vi "Handle Error.vi"(8 "error in (no error)":errorcluster, 11 "Sim Sensor Interface Actor in":refnum<class "Sim Sensor Interface Actor.lvclass">) -> (0 "error out":errorcluster, 2 "stop actor?":bool=TRUE, 3 "Sim Sensor Interface Actor out":refnum<class "Sim Sensor Interface Actor.lvclass">)   [LabVIEW 2022 SP3, in "Sim Sensor Interface Actor.lvlib" / "Sim Sensor Interface Actor.lvclass"]
doc: "(<B>Filename</B>: Actor Framework.lvlib:Actor.lvclass:Handle Error.vi)\n\nDefines how the actor handles an error that occurred while processing a message.\n\nBy default, this method does nothing except stop the actor. This method also treats error code 43 (coming from <B>error in</B>) as a sign that the actor shut down normally. In this situation, the Handle Error method does not return the error on <B>error out</B>, meaning the actor's caller will not receive it. All other error codes will be returned on <B>error out</B>.\n\nA descendant class may override this method to change this behavior."
uses:
  Sim Sensor Interface Actor.lvclass
  C:/Program Files/National Instruments/LabVIEW 2022/vi.lib/ActorFramework/Actor/Actor.lvclass
  Elevator Controller/Elevator Controller/States -Enum.ctl
  <vilib>/ActorFramework/Actor/Actor.lvclass/Actor.ctl
  Elevator Controller/Elevator Controller Messages/Centralize Error Msg/Centralize Error Msg.lvclass/Centralize Error Msg.ctl
  <vilib>/ActorFramework/Message Enqueuer/Message Enqueuer.lvclass/Message Enqueuer.ctl
  Elevator Controller/Elevator Controller Messages/Set State Msg/Set State Msg.lvclass/Set State Msg.ctl
  <vilib>/ActorFramework/Message Enqueuer/Enqueue.vi
  Elevator Controller/Elevator Controller Messages/Centralize Error Msg/Centralize Error Msg.lvclass
  C:/Program Files/National Instruments/LabVIEW 2022/vi.lib/ActorFramework/Message/Message.lvclass
  Elevator Controller/Elevator Controller Messages/Set State Msg/Set State Msg.lvclass
  <vilib>/ActorFramework/Message Priority Queue/Priority Enqueue.vi
  Abstract Sensor Interface Actor/Abstract Sensor Interface Actor/Abstract Sensor Interface Actor.lvclass
  Sim Sensor Interface Actor.lvclass/Sim Sensor Interface Actor.ctl
  <vilib>/ActorFramework/Actor/Actor.lvclass
  Elevator Controller/Elevator Controller/Elevator Controller.lvclass
  Incoming Messages/Set State Msg/Set State Msg.lvclass
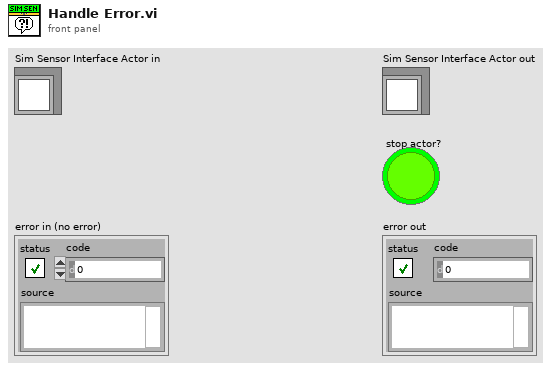
[diagram p1: front panel]
types:
  T1 = typedef "Elevator Controller.lvlib/Elevator Controller.lvclass/States -Enum.ctl" = enum16{"Initial State", "Wait for First Request", "Start and Move State", "Analysis State", "Continue Travel State", "Stop at Floor", "Open and Close Door Sequence", "No Request Remaining", "Emergency Call", "Terminate Process", ""}
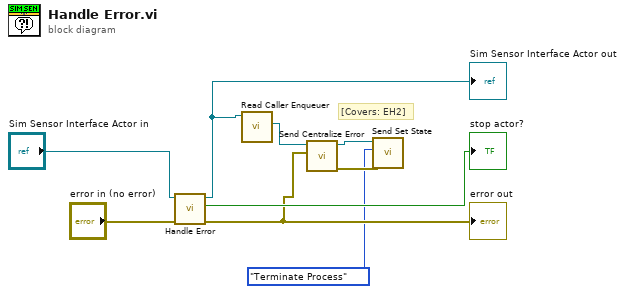
[diagram p0: block diagram]
diagram:
  # "[Covers: EH2]"
  n1 = call-parent "Handle Error.vi"("error in (no error)"="error in (no error)", "Actor in"="Sim Sensor Interface Actor in") -> ("error out"=w4:errorcluster, "stop actor?"=→"stop actor?":bool, "Actor out"=w5:refnum<class "Sim Sensor Interface Actor.lvclass">)  [unwired: 7 in]
  "Sim Sensor Interface Actor out" <- w5
  "error out" <- w4
  n2 = call <vilib>:"Read Caller Enqueuer.vi"("Actor"=w5) -> ("Caller Enqueuer"=w6:refnum<class "Message Enqueuer.lvclass">)  [unwired: 10 in]
  n3 = call "Send Centralize Error.vi"("Error"=w4, "Message Enqueuer"=w6) -> ("error out"=w2:errorcluster, "Message Enqueuer out"=w3:refnum<class "Message Enqueuer.lvclass">)  [unwired: 8 in]
  n4 = call "Send Set State.vi"("error in (no error)"=w2, "State"=States_-Enum."Terminate Process" ("Enum"), "Message Enqueuer"=w3) -> ()  [unwired: 7 in, 2 out]
